vi "myIP.vi"() -> (0 "My IP":string)   [LabVIEW 2015]
doc: "Gives in output the IP of the computer where is running."
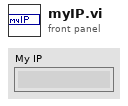
[diagram p1: front panel]
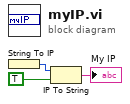
[diagram p0: block diagram]
diagram:
  n1 = String To IP() -> (0:w3:u32)  [unwired: 1 in]
  n2 = IP To String(1:TRUE ("dot notation? (F)"), 2:w3) -> (0:→"My IP":string)
